vi "PathPlanner_PathFinder_GetAllNeighbors.vi"(11 "GridPosition":T1) -> (3 "Neighbors":T1[](array[typedef]))   [LabVIEW 2019, in "PathPlanner24.lvlib"]
doc: "Internal function. Not to be used by end users."
uses:
  PathPlanner24.lvlib
  TypeDef/PathPlannerFinderGridPosition.ctl
  PathPlanner_PathFinder_Globals.vi
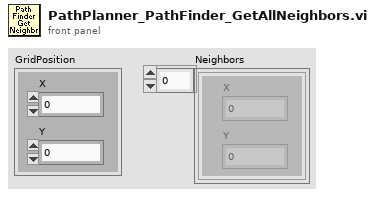
[diagram p1: front panel]
types:
  T1 = typedef "PathPlanner24.lvlib/PathPlannerFinderGridPosition.ctl" = cluster{"X":i32, "Y":i32}
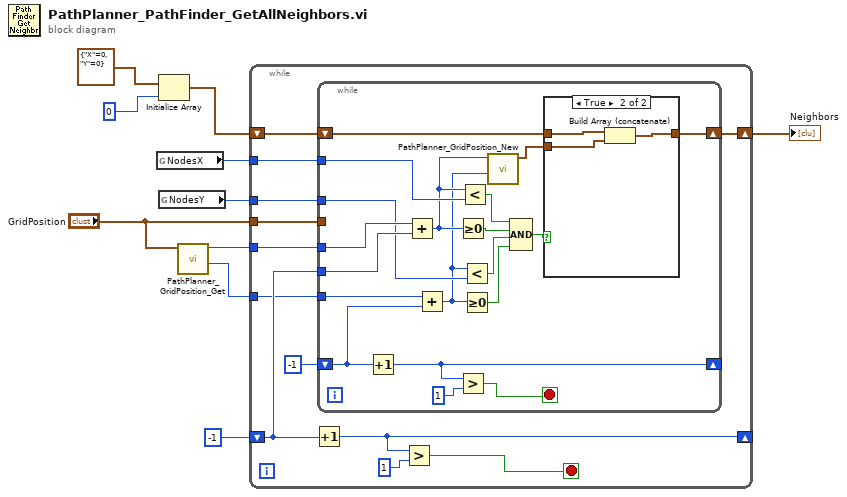
[diagram p0: block diagram]
diagram:
  n1 = global read "PathPlanner_PathFinder_Globals.vi" "NodesX"() -> (w5:i32)
  n2 = Initialize Array(T1 {"X"=0, "Y"=0} ("Neighbors"), 0 ("dimension size")) -> (w3:T1[])
  n3 = global read "PathPlanner_PathFinder_Globals.vi" "NodesY"() -> (w4:i32)
  n4 = call "PathPlanner_GridPosition_Get.vi"("GridPosition"="GridPosition") -> ("Int Y"=w6:i32, "Int X"=w7:i32)  [unwired: 9 in]
  n5 = while {
    shift-right: [w22] -> _
    shift-left: -1 ("dimension size") -> [w18]
    tunnel: w7 -> [w17]
    tunnel: w6 -> [w16]
    tunnel: w5 -> [w15]
    tunnel: w4 -> [w14]
    shift-right: [w11] -> w1
    shift-left: w3 -> [w13]
    tunnel: "GridPosition" -> [w12]
    stop <- w20 stop-if-true
    n6 = Increment(x=w18) -> (x+1=w22:i32)
    n7 = while {
      shift-right: [w39] -> _
      shift-left: -1 ("dimension size") -> [w36]
      tunnel: w18 -> [w38]
      tunnel: w17 -> [w37]
      tunnel: w16 -> [w35]
      tunnel: w15 -> [w34]
      tunnel: w14 -> [w33]
      shift-right: [w26] -> w11
      shift-left: w13 -> [w27]
      tunnel: w12 -> [_]
      stop <- w40 stop-if-true
      n8 = Increment(x=w36) -> (x+1=w39:i32)
      n9 = Add(x=w37, y=w38) -> (x+y=w24:i32)
      n10 = Add(x=w35, y=w36) -> (x+y=w23:i32)
      n11 = Greater Or Equal To 0?(x=w24) -> (x >= 0?=w31:bool)
      n12 = Greater?(x=w39, y=1) -> (0:w40:bool)
      n13 = Less?(x=w24, y=w34) -> (x < y?=w32:bool)
      n14 = Less?(x=w23, y=w33) -> (x < y?=w30:bool)
      n15 = Greater Or Equal To 0?(x=w23) -> (x >= 0?=w29:bool)
      n16 = call "PathPlanner_GridPosition_New.vi"("Int Y"=w23, "Int X"=w24) -> ("GridPosition"=w25:T1)  [unwired: 9 in]
      n17 = Compound Arithmetic op=AND(w32, w31, w30, w29) -> (w28:bool)
      n18 = case shown="True" w28 {
        tunnel: w27 -> [w42 w45]
        tunnel: w25 -> [_ w44]
        tunnel: [w42 w43] -> w26
        frame False {
        }
        frame True {
          n19 = Build Array (concatenate)(w45, w44) -> (w43:T1[])
        }
      }
    }
    n20 = Greater?(x=w22, y=1) -> (0:w20:bool)
  }
  "Neighbors" <- w1
